vi "DexRegisterEvent.vi"   [LabVIEW 2020]
doc: "Dynamically registers events for a network stream endpoint."
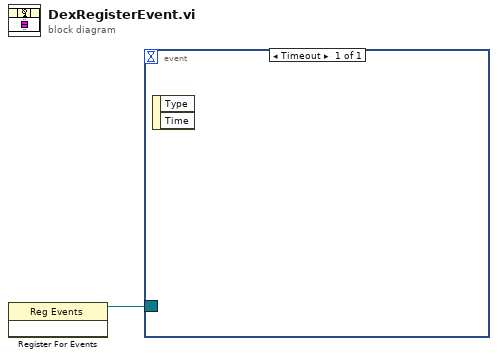
[diagram p0: block diagram]
diagram:
  n1 = register-events() -> (reference out=w1:refnum<event-registration>)  [unwired: 3 in, 1 out]
  n2 = event shown="[0] Timeout" {
    selector: w1 -> [_]
    dyn-events: _ -> [_]
    timeout: _ -> [_]
    event Timeout {
      n3 = event-data() -> ()  [unwired: 1 in, 2 out]
    }
  }
